vi "运维调试_采配水.vi"() -> ()   [LabVIEW 2016, in "PLC.lvlib"]
uses:
  PLC.lvlib
  <vilib>/Plasmionique/MB Master/MB_Master/MB_Master.lvclass
  <vilib>/Utility/miscctls.llb/LVPointTypeDef.ctl
  <vilib>/Plasmionique/MB Master/MB_Master_Serial/MB_Master_Serial.lvclass
  C:/Program Files (x86)/National Instruments/LabVIEW 2016/vi.lib/Plasmionique/MB Master/MB_Master/MB_Master.lvclass
  <vilib>/Plasmionique/MB Master/MB Master.lvlib
panel:
  out "R113":i16 caption="储水时间"
  out "R23":i16 caption="当前累计运行"
  out "R112":i16 caption="采配水运行"
  out "R22":i16
  in  "V8":bool
  out "R111":i16 caption="排液时间"
  out "通讯故障":bool
  out "R21":i16
  in  "V7":bool
  out "R20":i16
  in  "M1-2":bool
  in  "潜水泵工作模式":u16(ring) items=["泵1单泵单管路", "泵2单泵单管路", "双泵双管路"]
  out "X10":bool caption="废液报警"
  out "X9":bool caption="自来水检测"
  out "X8":bool caption="泵2过载报警"
  out "X7":bool caption="泵1过载报警"
  out "X6":bool caption="断电检测"
  out "X5":bool caption="开门检测"
  out "X4":bool caption="烟雾检测"
  out "X3":bool caption="漏水检测"
  out "X2":bool caption="进样检测"
  out "X1":bool
  out "X0":bool caption="采样池液位开关"
  out "Y12":bool caption="多参通电"
  out "R109":i16 caption="配水时间"
  out "集成报警信息":string
  out "R108":i16 caption="自来水进样超时设置"
  out "R107":i16 caption="采水池液位报警设置"
  out "R106":i16 caption="进样超时设置"
  out "R105":i16 caption="二级清洗时间"
  out "R104":i16 caption="一级清洗时间"
  out "R103":i16 caption="外部管路清洗时间"
  out "R102":i16 caption="静置沉淀时间"
  out "R101":i16 caption="内部管路润洗时间"
  out "R100":i16 caption="外部管路润洗时间"
  out "R2":i16
  out "R1":i16
  out "多列列表框":i32(listbox)
  out "R19":i16
  in  "V6":bool
  out "R18":i16
  in  "V5":bool
  out "R17":i16
  in  "V4":bool
  out "R16":i16
  in  "V3":bool
  out "R15":i16
  in  "V2":bool
  out "R14":i16
  in  "M2":bool
  out "R13":i16
  in  "V1":bool
  out "R12":i16
  in  "M1-1":bool
  in  "返回":bool
  in  "参数设置":bool
  in  "单步启动":bool
  in  "启动":bool
  in  "停止":bool
  # "S"
  # "次"
  # "次，清洗一次"
  # "S"
  # "S"
  # "S"
  # "S"
  # "S"
  # "S"
  # "S"
  # "S"
  # "S"
  # "S"
  # "S"
  # "单步计时："
  # "s"
  # "流程计时："
  # "s"
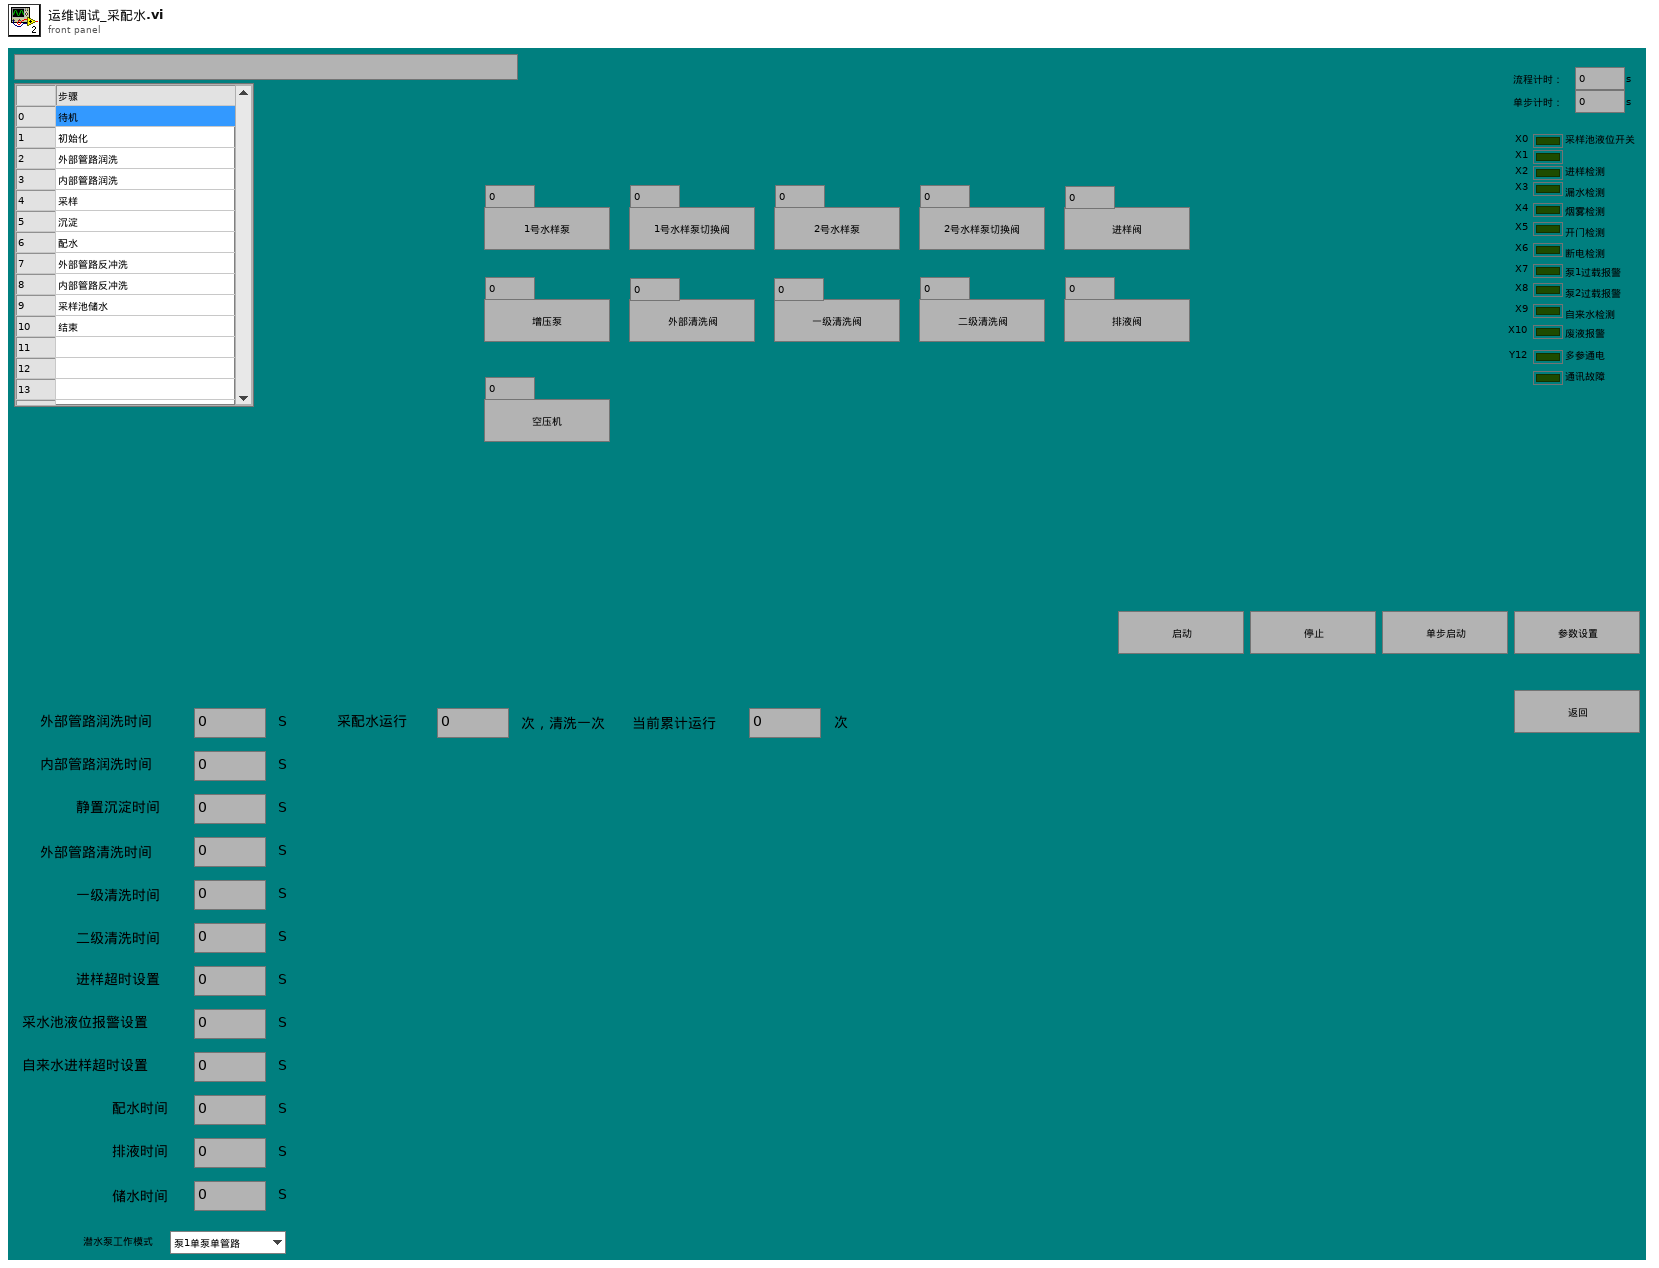
[diagram p1: front panel]
types:
  T1 = typedef "LVPointTypeDef.ctl" = cluster{"Horizontal":i16, "Vertical":i16}
  T2 = cluster{"命令":string, cluster{"starting address":u16, "holding register value":u16}}
  T3 = cluster{"命令":string, "数据":cluster{"starting address":u16, "holding register value":u16}}
  T4 = cluster{"命令":string, "数据":cluster{"starting address":u16, "holding register values":u16[]}}
  T5 = cluster{"命令":string, "data":cluster{"starting address":u16, "coil values":bool[]}}
  T6 = cluster{"测试模式":enum16{"正常测试", "集成干预"}, "参数启用":cluster{"氨氮":bool, "总磷总氮":bool, "CODMn":bool, "CODcr":bool, "多参数":bool, "超标留样":bool}}
  T7 = enum32{"Bad", "Idle", "Run top level", "Running"}
  T8 = cluster{"时间标识":timestamp, "设备":string, "日志信息":string}
  T9 = cluster{"R0":i16, "R1":i16, "R2":i16, "R3":i16, "R4":i16, "R5":i16, "R6":i16, "R7":i16, "R8":i16, "R9":i16, "R10":i16, "R11":i16, "R12":i16, "R13":i16, "R14":i16, "R15":i16, "R16":i16, "R17":i16, "R18":i16, "R19":i16, "R20":i16, "R21":i16, "R22":i16, "R23":i16, "R24":i16, "R25":i16, "R26":i16, "R27":i16, "R28":i16, "R29":i16, "R30":i16, "R31":i16, "R32":i16, "R33":i16, "R34":i16}
  T10 = cluster{"seconds since 1Jan1904":timestamp, "table输入":string, string, "table输入":string}
  T11 = cluster{"时间标识":timestamp, "设备":string, "日志信息":string, "流程参数":string}
  T12 = cluster{"baud rate (bps)":u32, "stop bits":u16, "parity":u16, "flow control":u16, "timeout":u32, "retries":i32}
  T13 = cluster{"starting address":u16, "holding register values":u16[]}
  T14 = cluster{"starting address":u16, "holding register value":u16}
  T15 = cluster{"starting address":u16, "coil values":bool[]}
  T16 = cluster{"Registers[0]":u16, "Registers[1]":u16, "Registers[2]":u16, "Registers[3]":u16, "Registers[4]":u16, "Registers[5]":u16, "Registers[6]":u16, "Registers[7]":u16, "Registers[8]":u16, "Registers[9]":u16, "Registers[10]":u16, "Registers[11]":u16, "Registers[12]":u16, "Registers[13]":u16, "Registers[14]":u16, "Registers[15]":u16, "Registers[16]":u16, "Registers[17]":u16, "Registers[18]":u16, "Registers[19]":u16, "Registers[20]":u16, "Registers[21]":u16, "Registers[22]":u16, "Registers[23]":u16, "Registers[24]":u16, "Registers[25]":u16, "Registers[26]":u16, "Registers[27]":u16, "Registers[28]":u16, "Registers[29]":u16, "Registers[30]":u16, "Registers[31]":u16, "Registers[32]":u16, "Registers[33]":u16, "Registers[34]":u16}
  T17 = cluster{"Registers[0]":u16, "Registers[1]":u16, "Registers[2]":u16, "Registers[3]":u16, "Registers[4]":u16, "Registers[5]":u16}
  T18 = cluster{"Registers[0]":u16, "Registers[1]":u16, "Registers[2]":u16, "Registers[3]":u16, "Registers[4]":u16, "Registers[5]":u16, "Registers[6]":u16, "Registers[7]":u16, "Registers[8]":u16, "Registers[9]":u16, "Registers[10]":u16, "Registers[11]":u16, "Registers[12]":u16, "Registers[13]":u16, "Registers[14]":u16, "Registers[15]":u16, "Registers[16]":u16, "Registers[17]":u16, "Registers[18]":u16, "Registers[19]":u16}
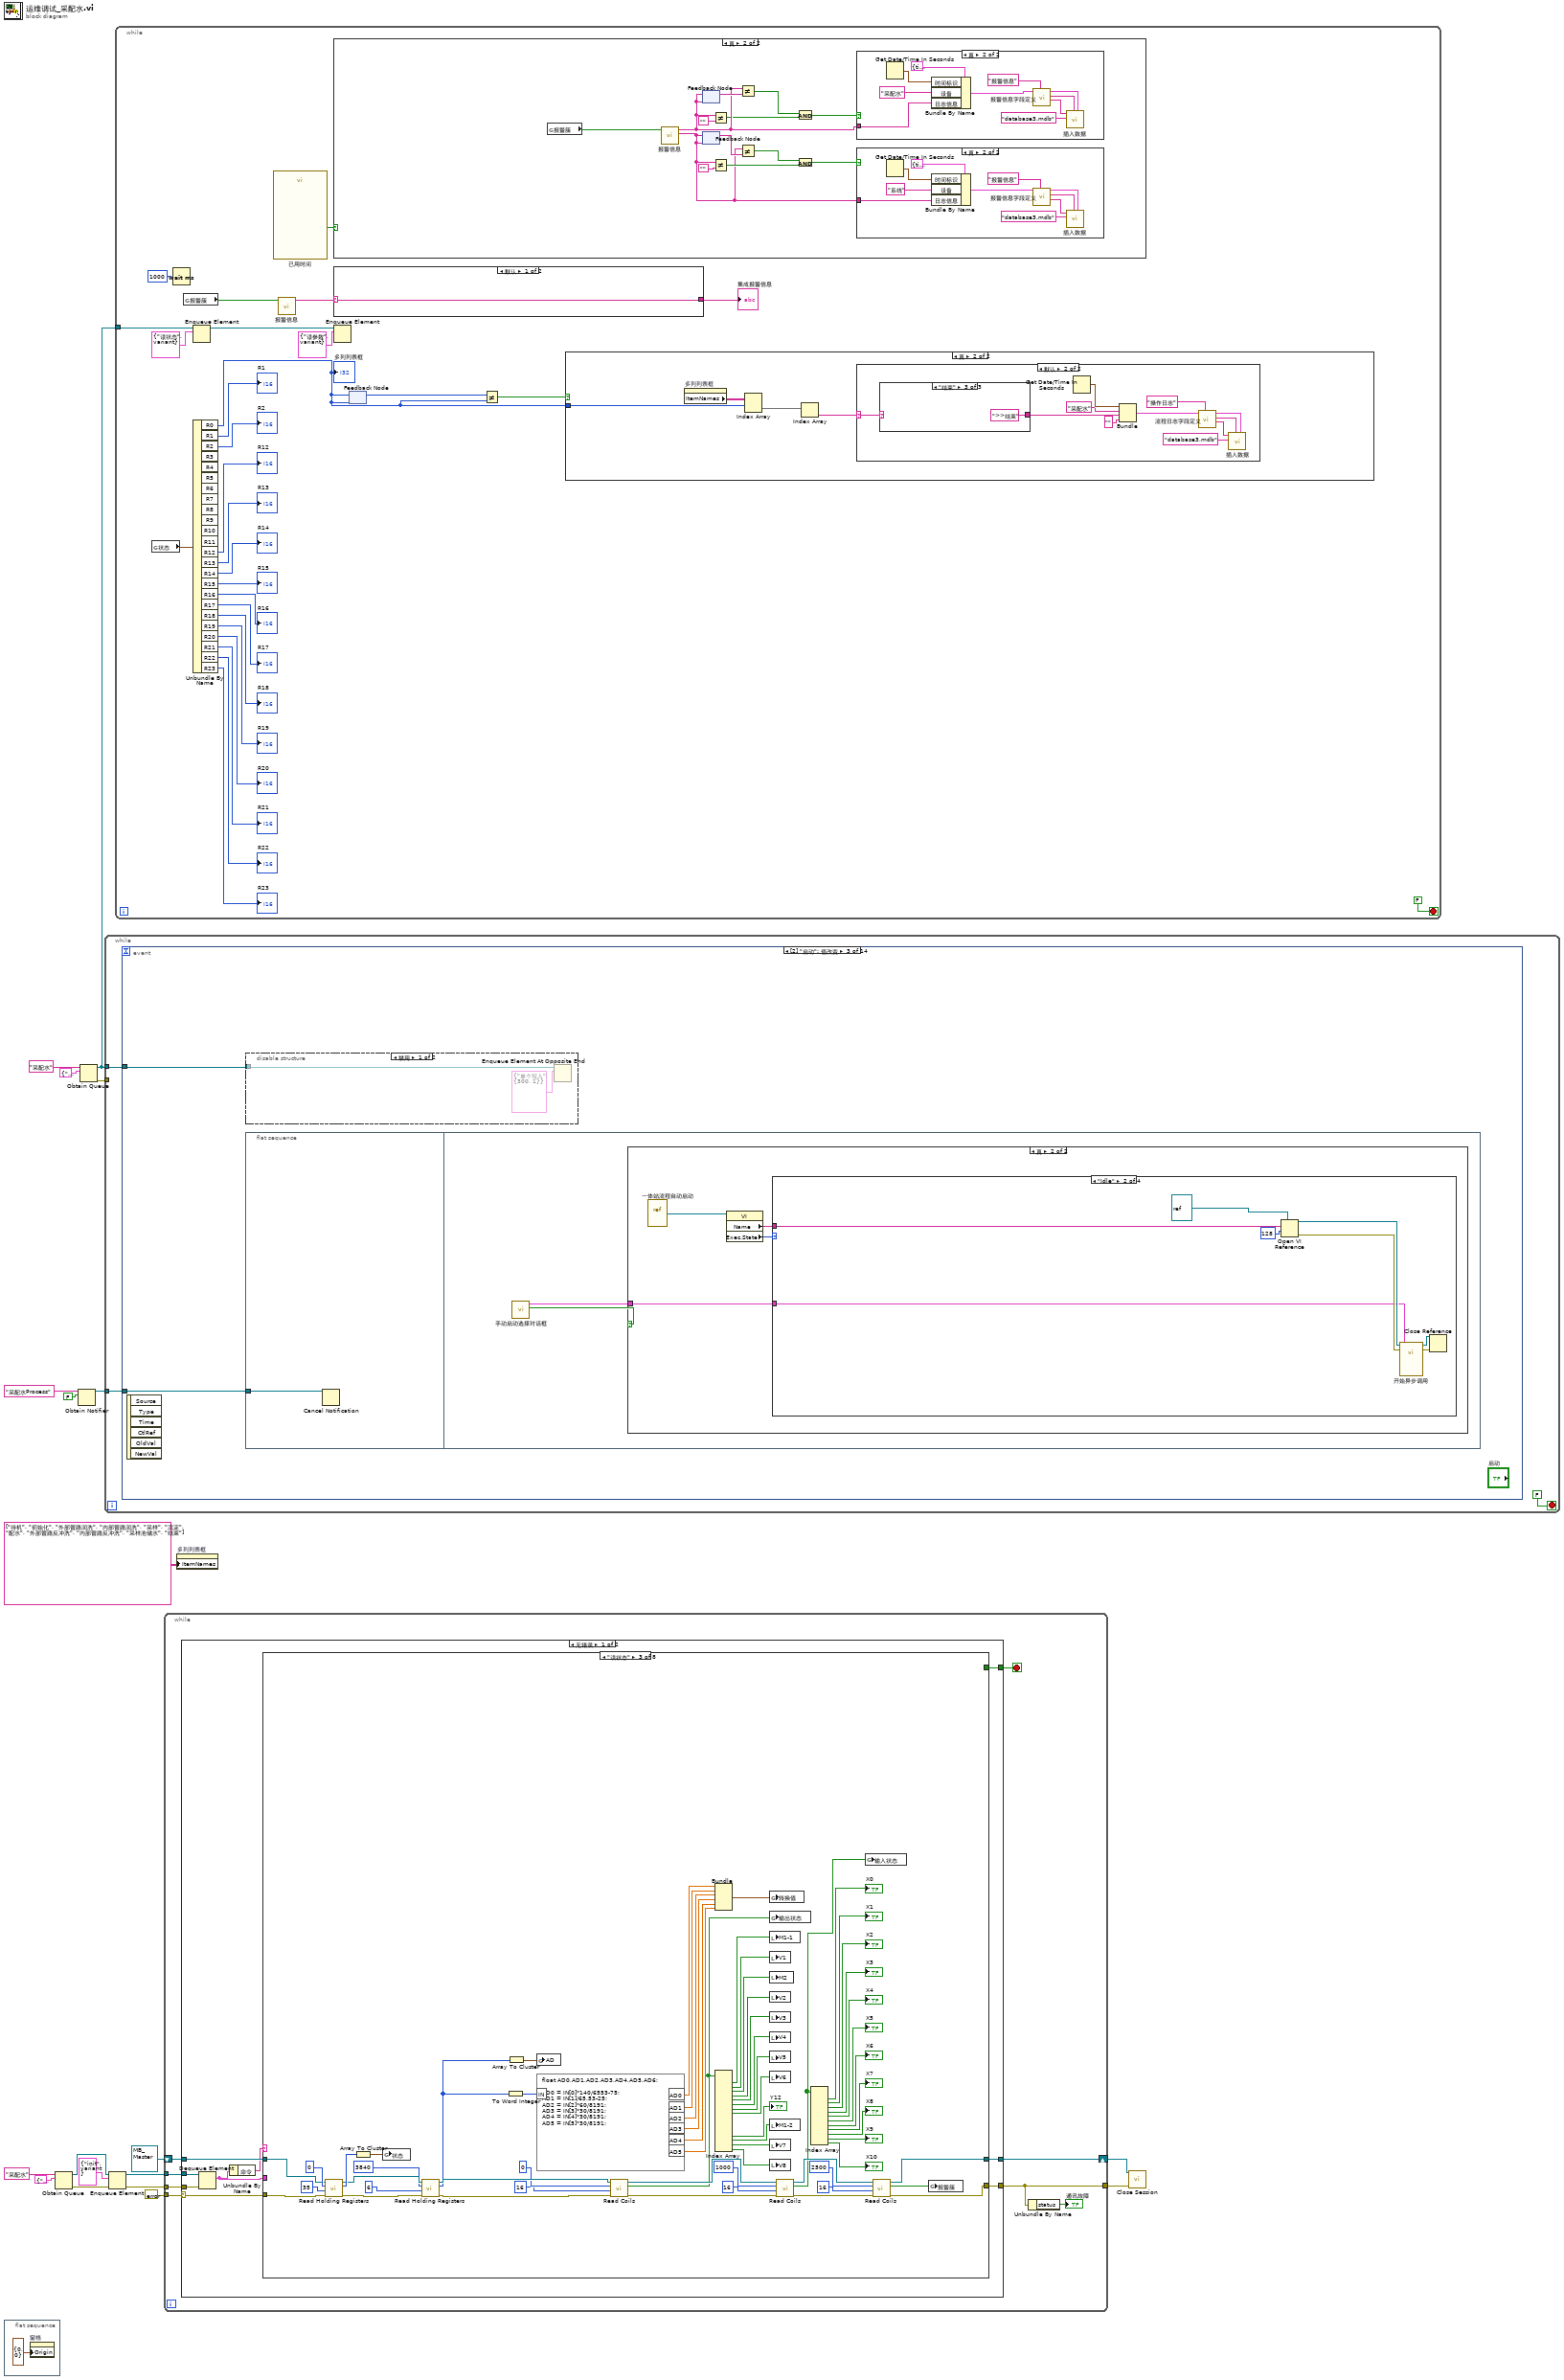
[diagram p0: block diagram]
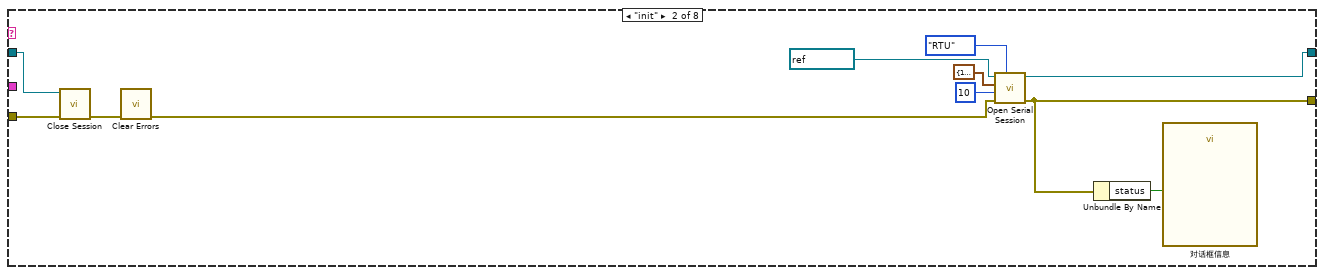
[diagram p3: hidden frame]
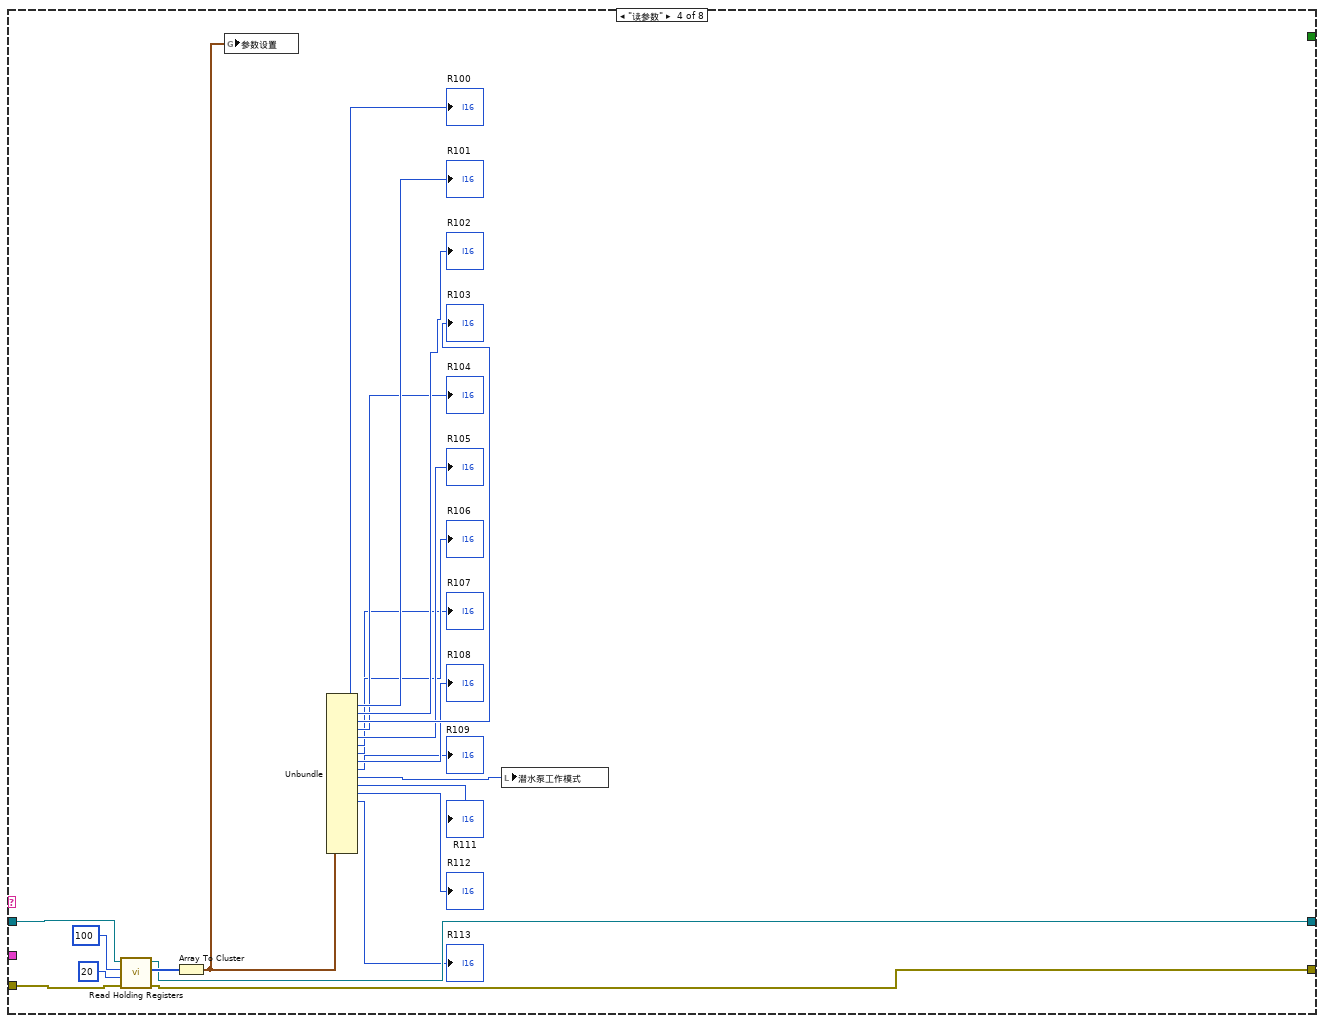
[diagram p4: hidden frame]
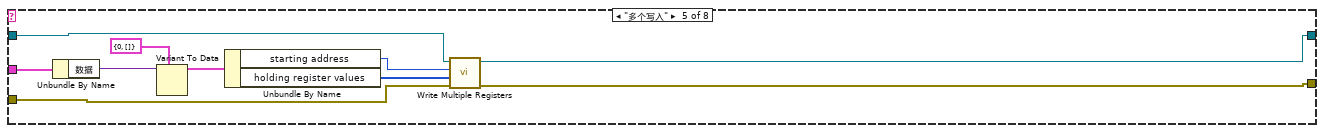
[diagram p5: hidden frame]
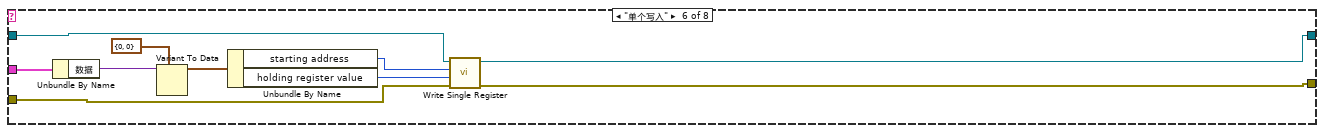
[diagram p6: hidden frame]
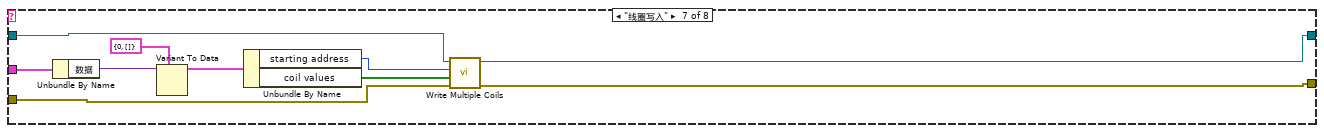
[diagram p7: hidden frame]
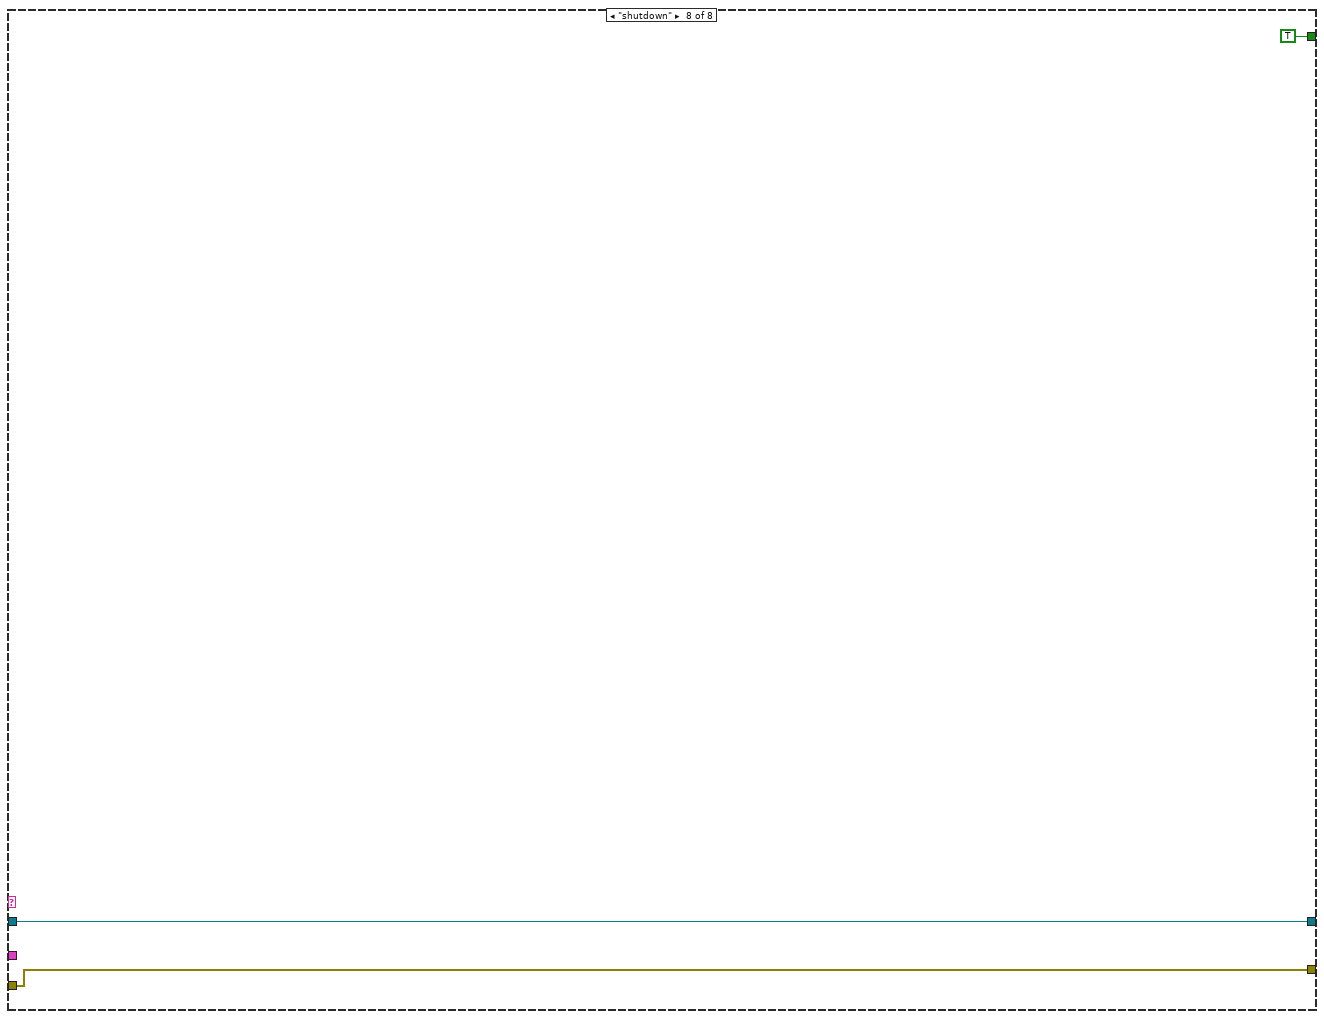
[diagram p8: hidden frame]
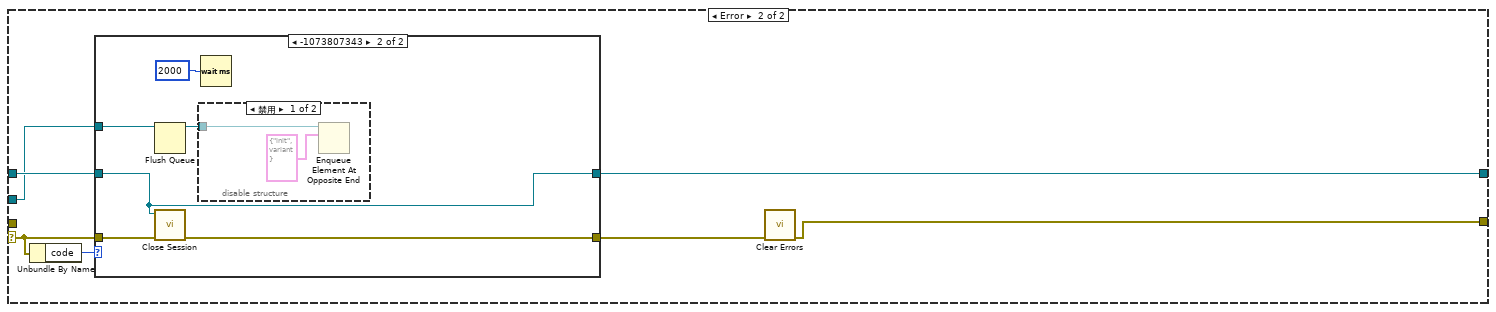
[diagram p9: hidden frame]
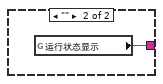
[diagram p15: hidden frame]
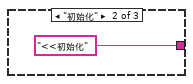
[diagram p19: hidden frame]
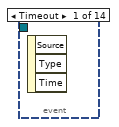
[diagram p20: hidden frame]
diagram:
  n1 = flat-sequence {
    frame #0 {
      n2 = property on="窗格" class="Pane"("Origin"=T1 {"Horizontal"=0, "Vertical"=0} ("原点")) -> ()  [unwired: 2 in, 2 out]
    }
  }
  n3 = Obtain Queue(name (unnamed)="采配水" ("名称（未命名）"), element data type=cluster{"命令":string, "数据":variant} {"命令"="", "数据"=variant}) -> (queue out=w9:refnum<queue>, error out=w8:errorcluster)  [unwired: 3 in, 1 out]
  n4 = Obtain Notifier(name (unnamed)="采配水Process" ("名称（未命名）"), notification data type=FALSE) -> (notifier out=w12:refnum<notifier>)  [unwired: 2 in, 2 out]
  n5 = Obtain Queue(name (unnamed)="采配水" ("名称（未命名）"), element data type=cluster{"命令":string, "数据":variant} {"命令"="", "数据"=variant}) -> (queue out=w16:refnum<queue>, error out=w17:errorcluster)  [unwired: 3 in, 1 out]
  n6 = while {
    tunnel: w16 -> [w22]
    tunnel: w17 -> [_]
    tunnel: w12 -> [w21]
    stop <- FALSE stop-if-true
    n7 = event shown="[2] \"启动\": 值改变" {
      selector: _ -> [_ _ _ _ _ _ _ _ _ _ _ _ _ _]
      dyn-events: _ -> [_ _ _ _ _ _ _ _ _ _ _ _ _ _]
      timeout: _ -> [_ _ _ _ _ _ _ _ _ _ _ _ _ _]
      tunnel: w22 -> [_ w26 w29 w51 w70 w73 _ _ _ _ w101 w103 w108 w113]
      tunnel: w21 -> [_ w25 w28 _ _ _ _ _ _ _ _ _ _ _]
      event Timeout {
        n8 = event-data() -> ()  [unwired: 1 in, 3 out]
      }
      event "停止": Value Change {
        n9 = event-data() -> ()  [unwired: 1 in, 6 out]
        n10 = Send Notification(notification=TRUE ("通知"), notifier=w25) -> ()  [unwired: 1 in, 2 out]
        n11 = Enqueue Element At Opposite End(queue=w26, element=T2 {"命令"="单个写入", {"starting address"=300, "holding register value"=2}} ("元素")) -> ()  [unwired: 2 in, 3 out]
      }
      event "启动": Value Change {
        n12 = event-data() -> ()  [unwired: 1 in, 6 out]
        n13 = disable-structure shown="禁用" {
          disable-tunnel: w29 -> [w47 _]
          frame Disabled {
            n14 = Enqueue Element At Opposite End(queue=w47, element=T2 {"命令"="单个写入", {"starting address"=300, "holding register value"=1}} ("元素")) -> ()  [unwired: 2 in, 3 out]
          }
          frame Enabled {
          }
        }
        n15 = flat-sequence {
          tunnel: w28 -> [w30]
          frame #0 {
            n16 = Cancel Notification(0:w30) -> ()  [unwired: 1 in, 3 out]
          }
          frame #1 {
            n17 = call "手动启动选择对话框.vi"() -> ("确定"=w31:bool, "参数"=w32:T6)  [unwired: 10 in]
            n18 = case shown="真" w31 {
              tunnel: w32 -> [_ w33]
              frame False {
              }
              frame True {
                n19 = vi-ref "一体站流程自动启动.vi"() -> (w36:refnum<vi>)
                n20 = property class="VI"(reference=w36) -> ("Name"=w35:string, "Exec.State"=w34:T7)  [unwired: 1 in, 2 out]
                n21 = case shown="\"Idle\"" w34 {
                  tunnel: w35 -> [_ w44 _ _]
                  tunnel: w33 -> [_ w38 _ _]
                  frame "Bad", Default {
                  }
                  frame "Idle" {
                    n22 = Open VI Reference(type specifier VI Refnum (for type only)=refnum<vi> refnum, vi path=w44, options=128 ("选项")) -> (vi reference=w42:refnum<vi>, error out=w40:errorcluster)  [unwired: 3 in]
                    n23 = call-by-ref "开始异步调用"(reference=w42, error in=w40, "参数"=w38) -> (reference out=w41:refnum<vi>, error out=w39:errorcluster)  [unwired: 11 in]
                    n24 = Close Reference(reference=w41, error in (no error)=w39) -> ()  [unwired: 1 out]
                  }
                  frame "Run top level" {
                  }
                  frame "Running" {
                    n25 = One Button Dialog(message="流程已经运行,无须重复启动" ("消息")) -> ()  [unwired: 1 in, 1 out]
                  }
                }
              }
            }
          }
        }
      }
      event "单步启动": Value Change {
        n26 = event-data() -> ()  [unwired: 1 in, 6 out]
        n27 = call "单步启动对话框.vi"() -> ("单步启动步骤输出"=w48:u16)  [unwired: 11 in]
        n28 = Bundle By Name(cluster=T3 {"命令"="单个写入", "数据"={"starting address"=301, "holding register value"=0}} ("元素"), "数据.holding register value"=w48) -> (w49:T3)
        n29 = Enqueue Element At Opposite End(queue=w51, element=w49) -> ()  [unwired: 2 in, 3 out]
      }
      event "R100", "R101", "R102", "R103", "R104", "R105", "R106", "R107", "R108", "R109", "潜水泵工作模式", "R111", "R112", "R113": Value Change {
        n30 = event-data() -> ()  [unwired: 1 in, 6 out]
        n31 = local read "R100"() -> (w65:i16)
        n32 = local read "R101"() -> (w64:i16)
        n33 = local read "R102"() -> (w63:i16)
        n34 = local read "R103"() -> (w62:i16)
        n35 = local read "R104"() -> (w61:i16)
        n36 = local read "R105"() -> (w60:i16)
        n37 = local read "R106"() -> (w59:i16)
        n38 = local read "R107"() -> (w58:i16)
        n39 = local read "R108"() -> (w57:i16)
        n40 = local read "R109"() -> (w56:i16)
        n41 = local read "R111"() -> (w54:i16)
        n42 = local read "R112"() -> (w53:i16)
        n43 = local read "R113"() -> (w52:i16)
        n44 = Build Array(w65, w64, w63, w62, w61, w60, w59, w58, w57, w56, "潜水泵工作模式", w54, w53, w52) -> (w66:u16[])
        n45 = Bundle By Name(cluster=T4 {"命令"="多个写入", "数据"={"starting address"=0, "holding register values"=[]}} ("元素"), "数据.starting address"=u16 100, "数据.holding register values"=w66) -> (w67:T4)
        n46 = Enqueue Element At Opposite End(queue=w70, element=w67) -> ()  [unwired: 2 in, 3 out]
      }
      event "R23": Value Change {
        n47 = event-data() -> ()  [unwired: 1 in, 6 out]
        n48 = local read "R23"() -> (w72:i16)
        n49 = Build Array(w72) -> (w71:i16[])
        n50 = Bundle By Name(cluster=T4 {"命令"="多个写入", "数据"={"starting address"=0, "holding register values"=[]}} ("元素"), "数据.starting address"=u16 23, "数据.holding register values"=w71) -> (w74:T4)
        n51 = Enqueue Element At Opposite End(queue=w73, element=w74) -> ()  [unwired: 2 in, 3 out]
      }
      event "R23": Mouse Down {
        n52 = event-data() -> ("CtlRef"=w79:refnum<vi>)  [unwired: 1 in, 7 out]
        n53 = Two Button Dialog(message="请确认是否更改，更改后将影响实际清洗频次" ("消息")) -> (T button?=w78:bool)  [unwired: 2 in]
        n54 = case shown="真" w78 {
          tunnel: w79 -> [_ w80]
          frame False {
          }
          frame True {
            n55 = property class="DigNum (严格)"(reference=w80) -> (reference out=w82:refnum<vi>, "Value"=w83:i16)  [unwired: 1 in, 1 out]
            n56 = call "数字键盘.vi"("OldNumber"=w83) -> ("NewNumber"=w81:sgl)
            n57 = property class="DigNum (严格)"(reference=w82, "Val(Sgnl)"=w81) -> ()  [unwired: 1 in, 2 out]
          }
        }
      }
      event "R100", "R101", "R102", "R103", "R104", "R105", "R106", "R107", "R108", "R109", "R111", "R112", "R113": Mouse Down {
        n58 = event-data() -> ("CtlRef"=w87:refnum<vi>)  [unwired: 1 in, 7 out]
        n59 = property class="DigNum (严格)"(reference=w87) -> (reference out=w85:refnum<vi>, "Value"=w86:i16)  [unwired: 1 in, 1 out]
        n60 = call "数字键盘.vi"("OldNumber"=w86) -> ("NewNumber"=w84:sgl)
        n61 = property class="DigNum (严格)"(reference=w85, "Val(Sgnl)"=w84) -> ()  [unwired: 1 in, 2 out]
      }
      event "参数设置": Value Change {
        n62 = event-data() -> ()  [unwired: 1 in, 6 out]
        n63 = property on="窗格" class="Pane"("Origin"=T1 {"Horizontal"=0, "Vertical"=628} ("原点")) -> ()  [unwired: 2 in, 2 out]
      }
      event "返回": Value Change {
        n64 = event-data() -> ()  [unwired: 1 in, 6 out]
        n65 = property on="窗格" class="Pane"("Origin"=T1 {"Horizontal"=0, "Vertical"=0} ("原点")) -> ()  [unwired: 2 in, 2 out]
      }
      event "M1-1", "V1", "M2", "V2", "V3", "V4", "V5", "V6": Value Change {
        n66 = event-data() -> ()  [unwired: 1 in, 6 out]
        n67 = Build Array("M1-1", "V1", "M2", "V2", "V3", "V4", "V5", "V6") -> (w90:bool[])
        n68 = Bundle By Name(cluster=T5 {"命令"="线圈写入", "data"={"starting address"=2400, "coil values"=[]}} ("元素"), "data.coil values"=w90) -> (w91:T5)
        n69 = Enqueue Element(queue=w101, element=w91) -> ()  [unwired: 2 in, 3 out]
      }
      event "M1-2": Value Change {
        n70 = event-data() -> ()  [unwired: 1 in, 6 out]
        n71 = Build Array("M1-2") -> (w104:bool[])
        n72 = Bundle By Name(cluster=T5 {"命令"="线圈写入", "data"={"starting address"=2413, "coil values"=[]}} ("元素"), "data.coil values"=w104) -> (w105:T5)
        n73 = Enqueue Element(queue=w103, element=w105) -> ()  [unwired: 2 in, 3 out]
      }
      event "V7": Value Change {
        n74 = event-data() -> ()  [unwired: 1 in, 6 out]
        n75 = Build Array("V7") -> (w109:bool[])
        n76 = Bundle By Name(cluster=T5 {"命令"="线圈写入", "data"={"starting address"=2414, "coil values"=[]}} ("元素"), "data.coil values"=w109) -> (w110:T5)
        n77 = Enqueue Element(queue=w108, element=w110) -> ()  [unwired: 2 in, 3 out]
      }
      event "V8": Value Change {
        n78 = event-data() -> ()  [unwired: 1 in, 6 out]
        n79 = Build Array("V8") -> (w114:bool[])
        n80 = Bundle By Name(cluster=T5 {"命令"="线圈写入", "data"={"starting address"=2415, "coil values"=[]}} ("元素"), "data.coil values"=w114) -> (w115:T5)
        n81 = Enqueue Element(queue=w113, element=w115) -> ()  [unwired: 2 in, 3 out]
      }
    }
  }
  n82 = Enqueue Element(queue=w9, element=cluster{"命令":string, "数据":variant} {"命令"="init", "数据"=variant} ("元素"), error in (no error)=w8) -> (queue out=w4:refnum<queue>, error out=w6:errorcluster)  [unwired: 1 in, 1 out]
  n83 = while {
    tunnel: w16 -> [w143]
    stop <- FALSE stop-if-true
    n84 = global read "采配水全局变量.vi" "状态"() -> (w141:T9)
    n85 = Wait (ms)(milliseconds to wait=u32 1000 ("等待时间（毫秒）")) -> ()  [unwired: 1 out]
    n86 = global read "采配水全局变量.vi" "报警簇"() -> (w129:bool[])
    n87 = Enqueue Element(queue=w143, element=cluster{"命令":string, "数据":variant} {"命令"="读状态", "数据"=variant} ("元素")) -> (queue out=w124:refnum<queue>)  [unwired: 2 in, 2 out]
    n88 = Unbundle By Name(w141) -> ("R0"=w122:i16, "R1"=→"R1":i16, "R2"=→"R2":i16, "R12"=→"R12":i16, "R13"=→"R13":i16, "R14"=→"R14":i16, "R15"=→"R15":i16, "R16"=→"R16":i16, "R17"=→"R17":i16, "R18"=→"R18":i16, "R19"=→"R19":i16, "R20"=→"R20":i16, "R21"=→"R21":i16, "R22"=→"R22":i16, "R23"=→"R23":i16)  [unwired: 9 out]
    "多列列表框" <- w122
    n89 = call "已用时间"() -> ("Time has Elapsed"=w127:bool)  [unwired: 12 in, 7 out]
    n90 = call "报警信息.vi"("报警簇"=w129) -> ("采配水报警信息"=w121:string)  [unwired: 9 in, 1 out]
    n91 = case shown="真" w127 {
      frame False {
      }
      frame True {
        n92 = global read "采配水全局变量.vi" "报警簇"() -> (w157:bool[])
        n93 = call "报警信息.vi"("报警簇"=w157) -> ("系统报警信息"=w146:string, "采配水报警信息"=w153:string)  [unwired: 9 in]
        n94 = feedback #1(w153) -> (w156:string)
        n95 = feedback-in #1(w153) -> ()
        n96 = feedback #2(w146) -> (w147:string)
        n97 = feedback-in #2(w146) -> ()
        n98 = Not Equal?(x=w153, y="") -> (x != y?=w151:bool)
        n99 = Not Equal?(x=w146, y="") -> (x != y?=w150:bool)
        n100 = Not Equal?(x=w153, y=w156) -> (x != y?=w155:bool)
        n101 = Not Equal?(x=w146, y=w147) -> (x != y?=w148:bool)
        n102 = And(x=w155, y=w151) -> (x .and. y?=w154:bool)
        n103 = And(x=w148, y=w150) -> (x .and. y?=w145:bool)
        n104 = case shown="真" w154 {
          tunnel: w153 -> [_ w168]
          frame False {
          }
          frame True {
            n105 = Get Date/Time In Seconds() -> (seconds since 1Jan1904=w170:timestamp)
            n106 = Bundle By Name(cluster=T8 {"时间标识"=timestamp(0 s since 1904-01-01), "设备"="", "日志信息"=""} ("data in"), "时间标识"=w170, "设备"="采配水", "日志信息"=w168) -> (w171:T8)
            n107 = call "报警信息字段定义.vi"("table输入"="报警信息", "data in"=w171) -> ("table输出"=w175:string, "columns"=w176:string[], "data out"=w177:T8)  [unwired: 7 in]
            n108 = call "插入数据.vi"("data"=w177, "columns"=w176, "database"="database3.mdb", "table"=w175) -> ()  [unwired: 7 in, 1 out]
          }
        }
        n109 = case shown="真" w145 {
          tunnel: w146 -> [_ w158]
          frame False {
          }
          frame True {
            n110 = Get Date/Time In Seconds() -> (seconds since 1Jan1904=w160:timestamp)
            n111 = Bundle By Name(cluster=T8 {"时间标识"=timestamp(0 s since 1904-01-01), "设备"="", "日志信息"=""} ("data in"), "时间标识"=w160, "设备"="系统", "日志信息"=w158) -> (w161:T8)
            n112 = call "报警信息字段定义.vi"("table输入"="报警信息", "data in"=w161) -> ("table输出"=w165:string, "columns"=w166:string[], "data out"=w167:T8)  [unwired: 7 in]
            n113 = call "插入数据.vi"("data"=w167, "columns"=w166, "database"="database3.mdb", "table"=w165) -> ()  [unwired: 7 in, 1 out]
          }
        }
      }
    }
    n114 = case shown="默认" w121 {
      selector: w121 -> [w178 _]
      tunnel: [w178 w179] -> w128
      frame Default {
      }
      frame "" {
        n115 = global read "采配水全局变量.vi" "运行状态显示"() -> (w179:string)
      }
    }
    "集成报警信息" <- w128
    n116 = Enqueue Element(queue=w124, element=cluster{"命令":string, "数据":variant} {"命令"="读参数", "数据"=variant} ("元素")) -> ()  [unwired: 2 in, 3 out]
    n117 = feedback-in #3(w122) -> ()
    n118 = feedback #3(w122) -> (w123:i16)
    n119 = Not Equal?(x=w123, y=w122) -> (x != y?=w130:bool)
    n120 = case shown="真" w130 {
      tunnel: w122 -> [_ w182]
      frame False {
      }
      frame True {
        n121 = property on="多列列表框" class="MCListbox (严格)"() -> ("ItemNames"=w183:string[][])  [unwired: 2 in, 2 out]
        n122 = Index Array(array=w183, index (row)=w182) -> (element=w181:string[])  [unwired: 1 in]
        n123 = Index Array(array=w181) -> (element=w180:string)  [unwired: 1 in]
        n124 = case shown="默认" w180 {
          selector: w180 -> [_ w185]
          frame "待机" {
          }
          frame Default {
            n125 = case shown="\"结束\"" w185 {
              selector: w185 -> [w195 _ _]
              tunnel: [w195 "<<初始化" ">>结束"] -> w184
              frame Default {
              }
              frame "初始化" {
              }
              frame "结束" {
              }
            }
            n126 = Get Date/Time In Seconds() -> (seconds since 1Jan1904=w189:timestamp)
            n127 = Bundle("seconds since 1Jan1904"=w189, "table输入"="采配水", w184, "table输入"="") -> (w187:T10)  [unwired: 1 in]
            n128 = call "流程日志字段定义.vi"("table输入"="操作日志", "data in"=w187) -> ("table输出"=w192:string, "columns"=w193:string[], "data out"=w194:T11)  [unwired: 7 in]
            n129 = call "插入数据.vi"("data"=w194, "columns"=w193, "database"="database3.mdb", "table"=w192) -> ()  [unwired: 7 in, 1 out]
          }
        }
      }
    }
  }
  n130 = while {
    tunnel: w4 -> [w202]
    tunnel: w6 -> [w201]
    shift-right: [w205] -> w1
    shift-left: refnum<class "MB_Master.lvclass"> refnum ("MB session in") -> [w204]
    tunnel: errorcluster {"status"=FALSE, "code"=0, "source"=""} ("error out") -> [w203]
    tunnel: [w199] -> w2
    stop <- w200 stop-if-true
    n131 = case shown="无错误" w203 {
      selector: w203 -> [w211 w347]
      tunnel: [w214 w346] -> w205
      tunnel: w204 -> [w213 w348]
      tunnel: [w212 w344] -> w199
      tunnel: w202 -> [w208 w343]
      tunnel: w201 -> [w207 _]
      tunnel: [w209 _] -> w200
      frame No Error {
        n132 = Dequeue Element(queue=w208, error in (no error)=w207) -> (element=w206:cluster{"命令":string, "数据":variant})  [unwired: 1 in, 3 out]
        n133 = Unbundle By Name(w206) -> ("命令"=w210:string)
        n134 = case shown="\"读状态\"" w210 {
          tunnel: [w216 w220 w257 w304 w316 w326 w336 w341] -> w214
          tunnel: w213 -> [w216 w224 w275 w309 w319 w329 w339 w341]
          tunnel: [w215 w222 w256 w303 w317 w327 w337 w340] -> w212
          tunnel: w211 -> [w215 w226 w278 w308 w318 w328 w338 w340]
          tunnel: [_ _ _ _ _ _ _ TRUE] -> w209
          tunnel: w206 -> [_ _ _ _ w315 w325 w335 _]
          frame "idle", Default {
          }
          frame "init" {
            n135 = call-dynamic "Close Session.vi"("error in (no error)"=w226, "MB session in"=w224) -> ("error out"=w225:errorcluster)  [unwired: 9 in]
            n136 = call <vilib>:"Clear Errors.vi"("error in (no error)"=w225) -> ("error out"=w223:errorcluster)  [unwired: 5 in, 1 out]
            n137 = call <vilib>:"Open Serial Session.vi"("Mode (RTU)"=enum16{"RTU", "ASCII"}."RTU", "Error in"=w223, "Slave ID"=u8 10, "Serial Config"=T12 {"baud rate (bps)"=115200, "stop bits"=10, "parity"=0, "flow control"=0, "timeout"=500, "retries"=1}, "VISA Resource"=refnum<visa-resource-name> "COM3" ("VISA resource name")) -> ("Error out"=w222:errorcluster, "MB_Serial session"=w220:refnum<class "MB_Master_Serial.lvclass">)  [unwired: 5 in]
            n138 = Unbundle By Name(w222) -> ("status"=w227:bool)
            n139 = call "对话框信息"("Enable"=w227) -> ()  [unwired: 9 in, 2 out]
          }
          frame "读状态" {
            n140 = call <vilib>:"Read Holding Registers.vi"("error in (no error)"=w278, "quantity"=u16 35 ("number of holding registers"), "starting address"=u16 0, "MB session in"=w275) -> ("error out"=w272:errorcluster, "Registers"=w274:u16[], "MB session out"=w273:refnum<class "MB_Master.lvclass">)  [unwired: 5 in]
            n141 = Array To Cluster(array=w274) -> (cluster=w279:T16)
            n142 = global write "采配水全局变量.vi" "状态"(w279) -> ()
            n143 = call <vilib>:"Read Holding Registers.vi"("error in (no error)"=w272, "quantity"=u16 6 ("number of holding registers"), "starting address"=u16 3840, "MB session in"=w273) -> ("error out"=w268:errorcluster, "Registers"=w232:u16[], "MB session out"=w269:refnum<class "MB_Master.lvclass">)  [unwired: 5 in]
            n144 = To Word Integer(number=w232) -> (16bit integer=w231:i16[])
            n145 = Array To Cluster(array=w232) -> (cluster=w287:T17)
            n146 = global write "采配水全局变量.vi" "AD"(w287) -> ()
            n147 = formula code="float AD0,AD1,AD2,AD3,AD4,AD5,AD6;\n\nAD0 = IN[0]*140/6553-75;\nAD1 = IN[1]/65.53-25;\nAD2 = IN[2]*60/8191;\nAD3 = IN[3]*30/8191;\nAD4 = IN[4]*30/8191;\nAD5 = IN[5]*30/8191;"("IN"=w231) -> ("AD0"=w285:dbl, "AD1"=w284:dbl, "AD2"=w283:dbl, "AD3"=w282:dbl, "AD4"=w281:dbl, "AD5"=w280:dbl)
            n148 = call <vilib>:"Read Coils.vi"("error in (no error)"=w268, "quantity"=u16 16 ("number of coils"), "starting address"=u16 0, "MB session in"=w269) -> ("error out"=w264:errorcluster, "Coils"=w230:bool[], "MB session out"=w265:refnum<class "MB_Master.lvclass">)  [unwired: 5 in]
            n149 = Bundle(w285, w284, w283, w282, w281, w280) -> (w286:cluster{dbl, dbl, dbl, dbl, dbl, dbl})  [unwired: 1 in]
            n150 = Index Array(array=w230) -> (element #1=w243:bool, element #2=w242:bool, element #3=w241:bool, element #4=w240:bool, element #5=w239:bool, element #6=w238:bool, element #7=w237:bool, element #8=w236:bool, element #13=→"Y12":bool, element #14=w235:bool, element #15=w234:bool, element #16=w233:bool)  [unwired: 16 in, 4 out]
            n151 = global write "采配水全局变量.vi" "转换值"(w286) -> ()
            n152 = global write "采配水全局变量.vi" "输出状态"(w230) -> ()
            n153 = local write "M1-1"(w243) -> ()
            n154 = local write "V1"(w242) -> ()
            n155 = local write "M2"(w241) -> ()
            n156 = local write "V2"(w240) -> ()
            n157 = local write "V3"(w239) -> ()
            n158 = local write "V4"(w238) -> ()
            n159 = local write "V5"(w237) -> ()
            n160 = local write "V6"(w236) -> ()
            n161 = local write "M1-2"(w235) -> ()
            n162 = local write "V7"(w234) -> ()
            n163 = local write "V8"(w233) -> ()
            n164 = call <vilib>:"Read Coils.vi"("error in (no error)"=w264, "quantity"=u16 16 ("number of coils"), "starting address"=u16 1000, "MB session in"=w265) -> ("error out"=w260:errorcluster, "Coils"=w229:bool[], "MB session out"=w261:refnum<class "MB_Master.lvclass">)  [unwired: 5 in]
            n165 = Index Array(array=w229) -> (element #1=→"X0":bool, element #2=→"X1":bool, element #3=→"X2":bool, element #4=→"X3":bool, element #5=→"X4":bool, element #6=→"X5":bool, element #7=→"X6":bool, element #8=→"X7":bool, element #9=→"X8":bool, element #10=→"X9":bool, element #11=→"X10":bool)  [unwired: 11 in]
            n166 = global write "采配水全局变量.vi" "输入状态"(w229) -> ()
            n167 = call <vilib>:"Read Coils.vi"("error in (no error)"=w260, "quantity"=u16 16 ("number of coils"), "starting address"=u16 2500, "MB session in"=w261) -> ("error out"=w256:errorcluster, "Coils"=w228:bool[], "MB session out"=w257:refnum<class "MB_Master.lvclass">)  [unwired: 5 in]
            n168 = global write "采配水全局变量.vi" "报警簇"(w228) -> ()
          }
          frame "读参数" {
            n169 = call <vilib>:"Read Holding Registers.vi"("error in (no error)"=w308, "quantity"=u16 20 ("number of holding registers"), "starting address"=u16 100, "MB session in"=w309) -> ("error out"=w303:errorcluster, "Registers"=w305:u16[], "MB session out"=w304:refnum<class "MB_Master.lvclass">)  [unwired: 5 in]
            n170 = Array To Cluster(array=w305) -> (cluster=w292:T18)
            n171 = global write "采配水全局变量.vi" "参数设置"(w292) -> ()
            n172 = Unbundle(w292) -> ("Registers[0]"=→"R100":u16, "Registers[1]"=→"R101":u16, "Registers[2]"=→"R102":u16, "Registers[3]"=→"R103":u16, "Registers[4]"=→"R104":u16, "Registers[5]"=→"R105":u16, "Registers[6]"=→"R106":u16, "Registers[7]"=→"R107":u16, "Registers[8]"=→"R108":u16, "Registers[9]"=→"R109":u16, "Registers[10]"=w291:u16, "Registers[11]"=→"R111":u16, "Registers[12]"=→"R112":u16, "Registers[13]"=→"R113":u16)  [unwired: 6 out]
            n173 = local write "潜水泵工作模式"(w291) -> ()
          }
          frame "多个写入" {
            n174 = Unbundle By Name(w315) -> ("数据"=w314:variant)
            n175 = Variant To Data(type=T13 {"starting address"=0, "holding register values"=[]}, Variant=w314) -> (data=w312:T13)  [unwired: 1 in, 1 out]
            n176 = Unbundle By Name(w312) -> ("starting address"=w311:u16, "holding register values"=w310:u16[])
            n177 = call <vilib>:"Write Multiple Registers.vi"("error in (no error)"=w318, "values"=w310, "starting address"=w311, "MB session in"=w319) -> ("error out"=w317:errorcluster, "MB session out"=w316:refnum<class "MB_Master.lvclass">)  [unwired: 6 in]
          }
          frame "单个写入" {
            n178 = Unbundle By Name(w325) -> ("数据"=w324:variant)
            n179 = Variant To Data(type=T14 {"starting address"=0, "holding register value"=0}, Variant=w324) -> (data=w322:T14)  [unwired: 1 in, 1 out]
            n180 = Unbundle By Name(w322) -> ("starting address"=w321:u16, "holding register value"=w320:u16)
            n181 = call <vilib>:"Write Single Register.vi"("error in (no error)"=w328, "value"=w320, "address"=w321, "MB session in"=w329) -> ("error out"=w327:errorcluster, "MB session out"=w326:refnum<class "MB_Master.lvclass">)  [unwired: 6 in]
          }
          frame "线圈写入" {
            n182 = Unbundle By Name(w335) -> ("数据"=w334:variant)
            n183 = Variant To Data(type=T15 {"starting address"=0, "coil values"=[]}, Variant=w334) -> (data=w332:T15)  [unwired: 1 in, 1 out]
            n184 = Unbundle By Name(w332) -> ("starting address"=w331:u16, "coil values"=w330:bool[])
            n185 = call <vilib>:"Write Multiple Coils.vi"("error in (no error)"=w338, "values"=w330, "starting address"=w331, "MB session in"=w339) -> ("error out"=w337:errorcluster, "MB session out"=w336:refnum<class "MB_Master.lvclass">)  [unwired: 6 in]
          }
          frame "shutdown" {
          }
        }
      }
      frame Error {
        n186 = Unbundle By Name(w347) -> ("code"=w349:i32)
        n187 = case shown="-1073807343" w349 {
          tunnel: w348 -> [w351 w355]
          tunnel: w347 -> [w350 w357]
          tunnel: [w350 w356] -> w345
          tunnel: [w351 w355] -> w346
          tunnel: w343 -> [_ w354]
          frame Default {
          }
          frame -1073807343 {
            n188 = Flush Queue(queue=w354) -> (queue out=w353:refnum<queue>)  [unwired: 1 in, 2 out]
            n189 = call-dynamic "Close Session.vi"("error in (no error)"=w357, "MB session in"=w355) -> ("error out"=w356:errorcluster)  [unwired: 9 in]
            n190 = disable-structure shown="禁用" {
              disable-tunnel: w353 -> [w358 _]
              frame Disabled {
                n191 = Enqueue Element At Opposite End(queue=w358, element=cluster{"命令":string, "数据":variant} {"命令"="init", "数据"=variant} ("元素")) -> ()  [unwired: 2 in, 3 out]
              }
              frame Enabled {
              }
            }
            n192 = Wait (ms)(milliseconds to wait=u32 2000 ("等待时间（毫秒）")) -> ()  [unwired: 1 out]
          }
        }
        n193 = call <vilib>:"Clear Errors.vi"("error in (no error)"=w345) -> ("error out"=w344:errorcluster)  [unwired: 5 in, 1 out]
      }
    }
    n194 = Unbundle By Name(w199) -> ("status"=→"通讯故障":bool)
  }
  n195 = property on="多列列表框" class="MCListbox (严格)"("ItemNames"=string[][] [["待机"], ["初始化"], ["外部管路润洗"], ["内部管路润洗"], ["采样"], ["沉淀"], ["配水"], ["外部管路反冲洗"], ["内部管路反冲洗"], ["采样池储水"], ["结束"]] ("项名")) -> ()  [unwired: 2 in, 2 out]
  n196 = call-dynamic "Close Session.vi"("error in (no error)"=w2, "MB session in"=w1) -> ()  [unwired: 9 in, 1 out]
